vi "Bin Nanotimes in Pixel.vi"(4 "Nanotime Bin Step":dbl, 6 "# Nanotime Bins":i32, 8 "Error In":errorcluster, 9 "# Pixels X":i32, 10 "Pixel Boundary Indices":i32[](array[numeric]), 11 "Nanotimes":u32[](array[numeric])) -> (0 "Error Out":errorcluster, 3 "Gate Lines":u16[][](array[numeric]))   [LabVIEW 2021, in "PTU Files.lvlib"]
uses:
  PTU Files.lvlib
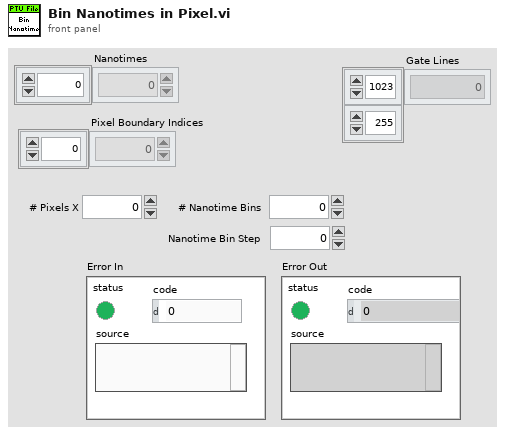
[diagram p1: front panel]
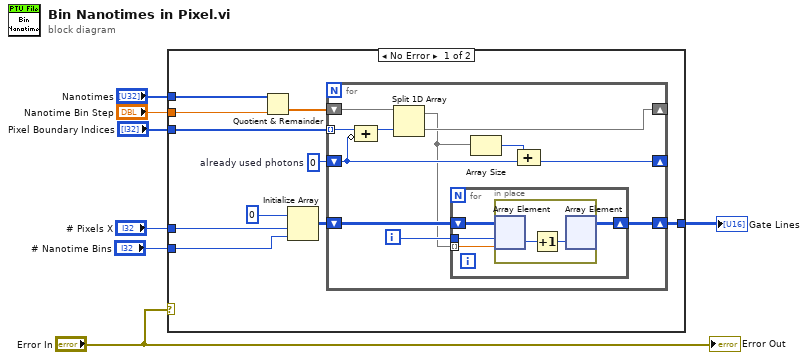
[diagram p0: block diagram]
diagram:
  n1 = case shown="No Error" "Error In" {
    tunnel: "Nanotimes" -> [w17 _]
    tunnel: "Nanotime Bin Step" -> [w16 _]
    tunnel: "# Pixels X" -> [w15 _]
    tunnel: [w12 _] -> w4
    tunnel: "# Nanotime Bins" -> [w10 _]
    tunnel: "Pixel Boundary Indices" -> [w9 _]
    frame No Error {
      w8 = u64 0  # already used photons
      n2 = Quotient & Remainder(x=w17, y=w16) -> (floor(x/y)=w11:dbl[])  [unwired: 1 out]
      n3 = Initialize Array(u16 0 ("Nanotime Bins"), w15, w10) -> (w13:u16[][])
      n4 = for {
        shift-right: [w25] -> w12
        shift-left: w13 -> [w28]
        shift-right: [w22] -> _
        shift-left: w11 -> [w27]
        tunnel: w9 -> [w26] mode=indexing
        shift-right: [w21] -> _
        shift-left: w8 -> [w19]
        i -> [w24]
        n5 = Compound Arithmetic op=ADD(w26, invert w19) -> (w20:u64)
        n6 = Split 1D Array(array=w27, index=w20) -> (first subarray=w18:dbl[], second subarray=w22:dbl[])
        n7 = for {
          tunnel: w24 -> [w30]
          shift-right: [w31] -> w25
          shift-left: w28 -> [w32]
          tunnel: w18 -> [w29] mode=indexing
          n8 = in-place {
            n9 = in-place-array #1(w32, w30, w29) -> (w34:u16)
            n10 = Increment(x=w34) -> (x+1=w33:u16)
            n11 = in-place-array #1(w33) -> (w31:u16[][])  [unwired: 2 out]
          }
        }
        n12 = Array Size(array=w18) -> (size(s)=w23:i32)
        n13 = Compound Arithmetic op=ADD(w23, w19) -> (w21:u64)
      }
    }
    frame Error {
    }
  }
  "Gate Lines" <- w4
  "Error Out" <- "Error In"
